vi "ConfFilterTest Main.vi"(8 "error in (no error)":errorcluster, 11 "Main Display in":refnum<class "Main Display.lvclass">) -> (0 "error out":errorcluster, 2 "Filter Name Array":string[](array[string]))   [LabVIEW 2016, in "Assert API Components.lvlib" / "Assert Display.lvlib" / "Main Display.lvlib" / "Main Display.lvclass"]
uses:
  Main Display.lvclass
  Assert API Components/Filter Configurations/Base Filter.lvclass
  Assert API Components/Filter Configurations/Base Filter.lvclass/Base Filter.ctl
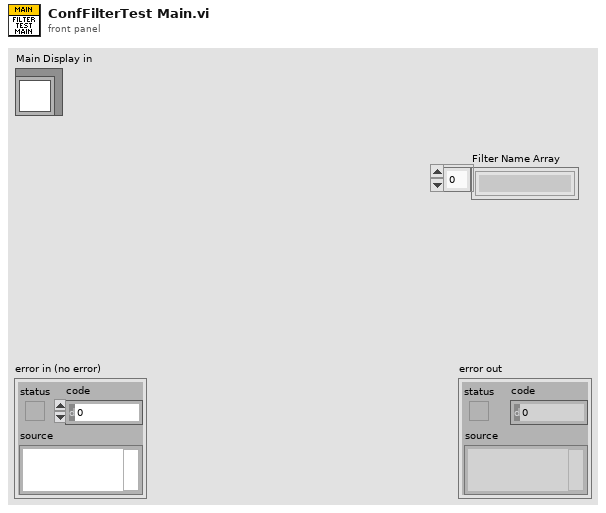
[diagram p1: front panel]
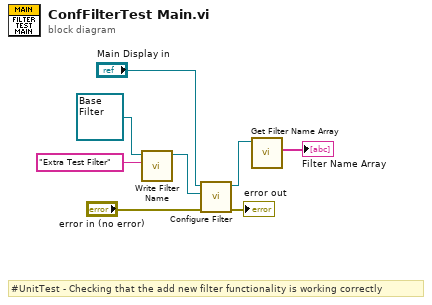
[diagram p0: block diagram]
diagram:
  # "#UnitTest - Checking that the add new filter functionality is working correctly"
  n1 = call "Write Filter Name.vi"("Filter Name"="Extra Test Filter", "Base Filter in"=refnum<class "Base Filter.lvclass"> refnum ("Assert API Components.lvlib:Base Filter.lvclass")) -> ("Base Filter out"=w5:refnum<class "Base Filter.lvclass">)  [unwired: 9 in]
  n2 = call "Configure Filter.vi"("error in (no error)"="error in (no error)", "New Filter"=w5, "Main Display in"="Main Display in") -> ("error out"=→"error out":errorcluster, "Main Display out"=w4:refnum<class "Main Display.lvclass">)  [unwired: 7 in]
  n3 = call "Get Filter Name Array.vi"("Main Display in"=w4) -> ("Filter Name Array"=→"Filter Name Array":string[])  [unwired: 10 in]
